vi "Read Exception Status.vi"(8 "error in (no error)":errorcluster, 11 "Modbus slave in":refnum<class "Modbus Slave.lvclass">) -> (0 "error out":errorcluster, 2 "exception status":u8, 3 "Modbus slave out":refnum<class "Modbus Slave.lvclass">)   [LabVIEW 2015, in "Modbus Slave.lvclass"]
doc: "Returns the exception status of a Modbus slave. The exception status is a set of eight status bits. Each status bit stands for an exception."
uses:
  <vilib>/Modbus/slave/Modbus Slave.lvclass
  <vilib>/Modbus/slave/Modbus Slave.lvclass/Modbus Slave.ctl
  <vilib>/Modbus/subvis/Data and Functions/Device Data Model/Device Data Model.lvclass
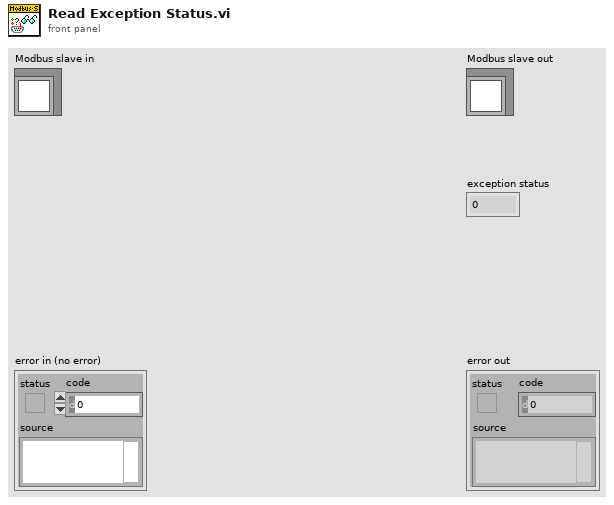
[diagram p1: front panel]
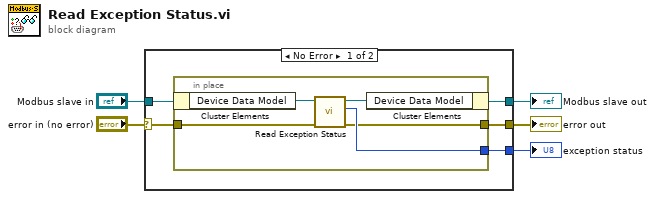
[diagram p0: block diagram]
diagram:
  n1 = case shown="No Error" "error in (no error)" {
    selector: "error in (no error)" -> [w6 w16]
    tunnel: "Modbus slave in" -> [w10 w17]
    tunnel: [w9 w17] -> w4
    tunnel: [w8 w16] -> w3
    tunnel: [w7 _] -> w2
    frame No Error {
      n2 = in-place {
        in-place-border: [w15] -> w7
        in-place-border: [w14] -> w8
        in-place-border: w6 -> [w13]
        n3 = in-place-cluster #1(w10) -> ("Device Data Model"=w12:refnum<class "Device Data Model.lvclass">)
        n4 = call-dynamic "Read Exception Status.vi"("error in (no error)"=w13, "device data model in"=w12) -> ("error out"=w14:errorcluster, "exception status"=w15:u8, "device data model out"=w11:refnum<class "Device Data Model.lvclass">)  [unwired: 7 in]
        n5 = in-place-cluster #1("Device Data Model"=w11) -> (w9:refnum<class "Modbus Slave.lvclass">)
      }
    }
    frame Error {
    }
  }
  "error out" <- w3
  "Modbus slave out" <- w4
  "exception status" <- w2
